vi "z_stack_waveform_Sunyee.vi"() -> ()   [LabVIEW 2018]
uses:
  <resource>/objmgr/daqmx.rc
  <vilib>/Utility/error.llb/DialogType.ctl
  <vilib>/DAQmx/create/channels.llb/DAQmx Create Channel (AO-Voltage-Basic).vi
  <vilib>/DAQmx/configure/timing.llb/DAQmx Timing (Sample Clock).vi
  <vilib>/Waveform/WDTOps.llb/WDT Append Waveforms DBL.vi
  <vilib>/DAQmx/write.llb/DAQmx Write (Analog 1D Wfm NChan NSamp).vi
  <vilib>/DAQmx/write.llb/DAQmx Write (Digital 1D Wfm NChan NSamp).vi
  <vilib>/DAQmx/configure/trigger.llb/DAQmx Start Trigger (Time).vi
  <vilib>/DAQmx/create/channels.llb/DAQmx Create Channel (DO-Digital Output).vi
  <vilib>/DAQmx/configure/trigger.llb/DAQmx Start Trigger (Digital Edge).vi
panel:
  in  "Line(s)":tag="Dev1/port0/line0:7"
  in  "Stop 2":bool
  in  "Trigger Type":T1(tab)
  in  "Edge":i32(ring)=10280 items=["Rising"=10280, "Falling"=10171]
  in  "Digital Trigger Source":tag="PFI1"
  in  "When":timestamp
  in  "Select Time\nManually":bool
  in  "Number of Samples":i32=1000
  in  "Sample Rate 2":dbl=1000.0
  in  "Sample Clock Source 2":tag="PFI0"
  out "Actual Sample Rate 2":dbl=1000.0 format="%0.2f"
  out "Waveform Graph 3":waveform(dbl)(graph)
  out "Waveform Graph 2":waveform(dbl)(graph)
  out "Waveform Graph":waveform(dbl)[](graph)
  in  "Stop":bool
  in  "Sample Rate":dbl=50000.0
  in  "Sample Clock Source":tag="OnboardClock"
  in  "Max Voltage":dbl=10.0
  in  "Min Voltage":dbl=-10.0
  in  "Physical Channel(s)":tag="PXI1Slot4_2/ao0:7"
  out "Actual Sample Rate":dbl=1000.0 format="%0.2f"
  # "To configure and use a start trigger you must have the necessary tab selected above.  Not all hardware supports triggering--refer to your device documentation for more info."
  # "If time is not manually set, task will begin after 10 seconds"
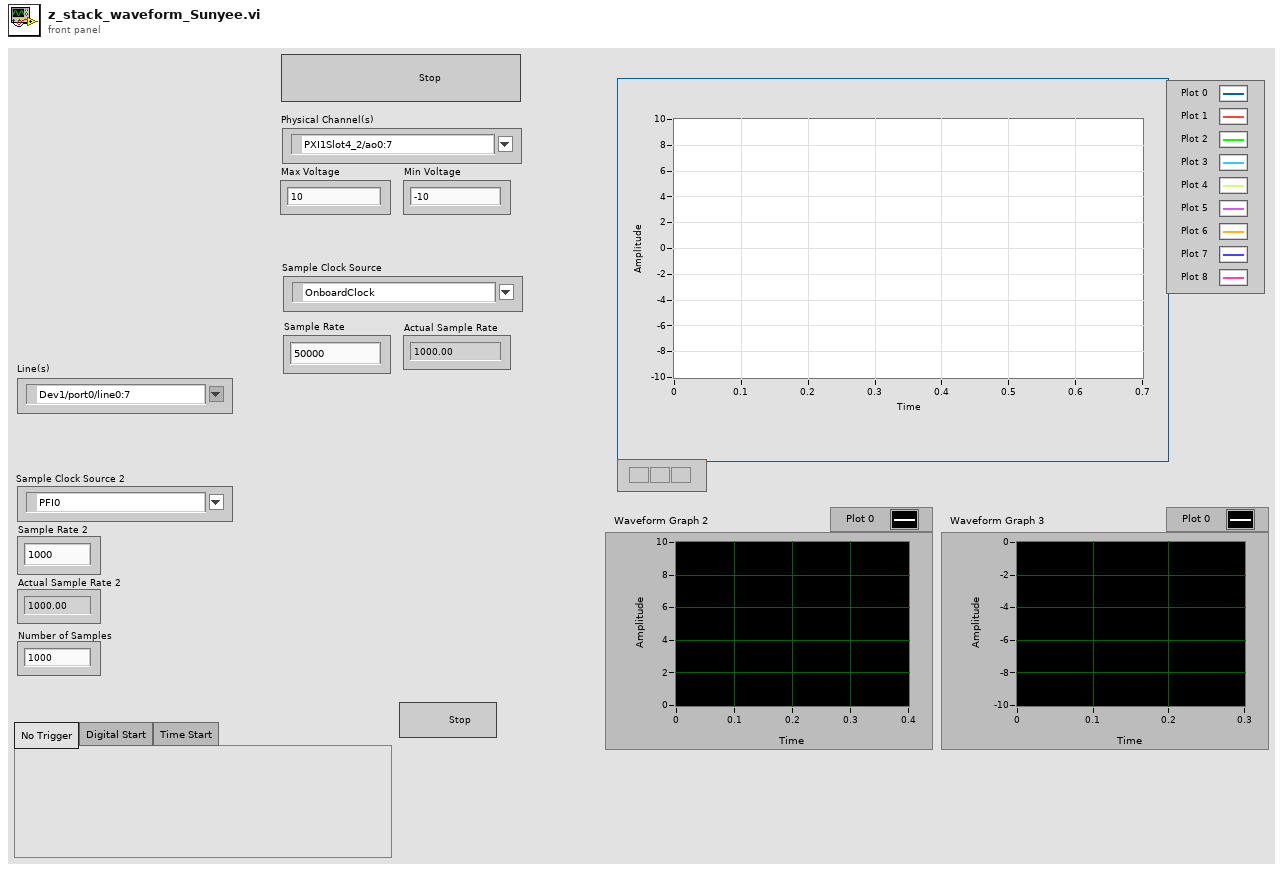
[diagram p1: front panel]
types:
  T1 = enum32{"No Trigger", "Digital Start", "Time Start"}
  T2 = typedef "DialogType.ctl" = u16
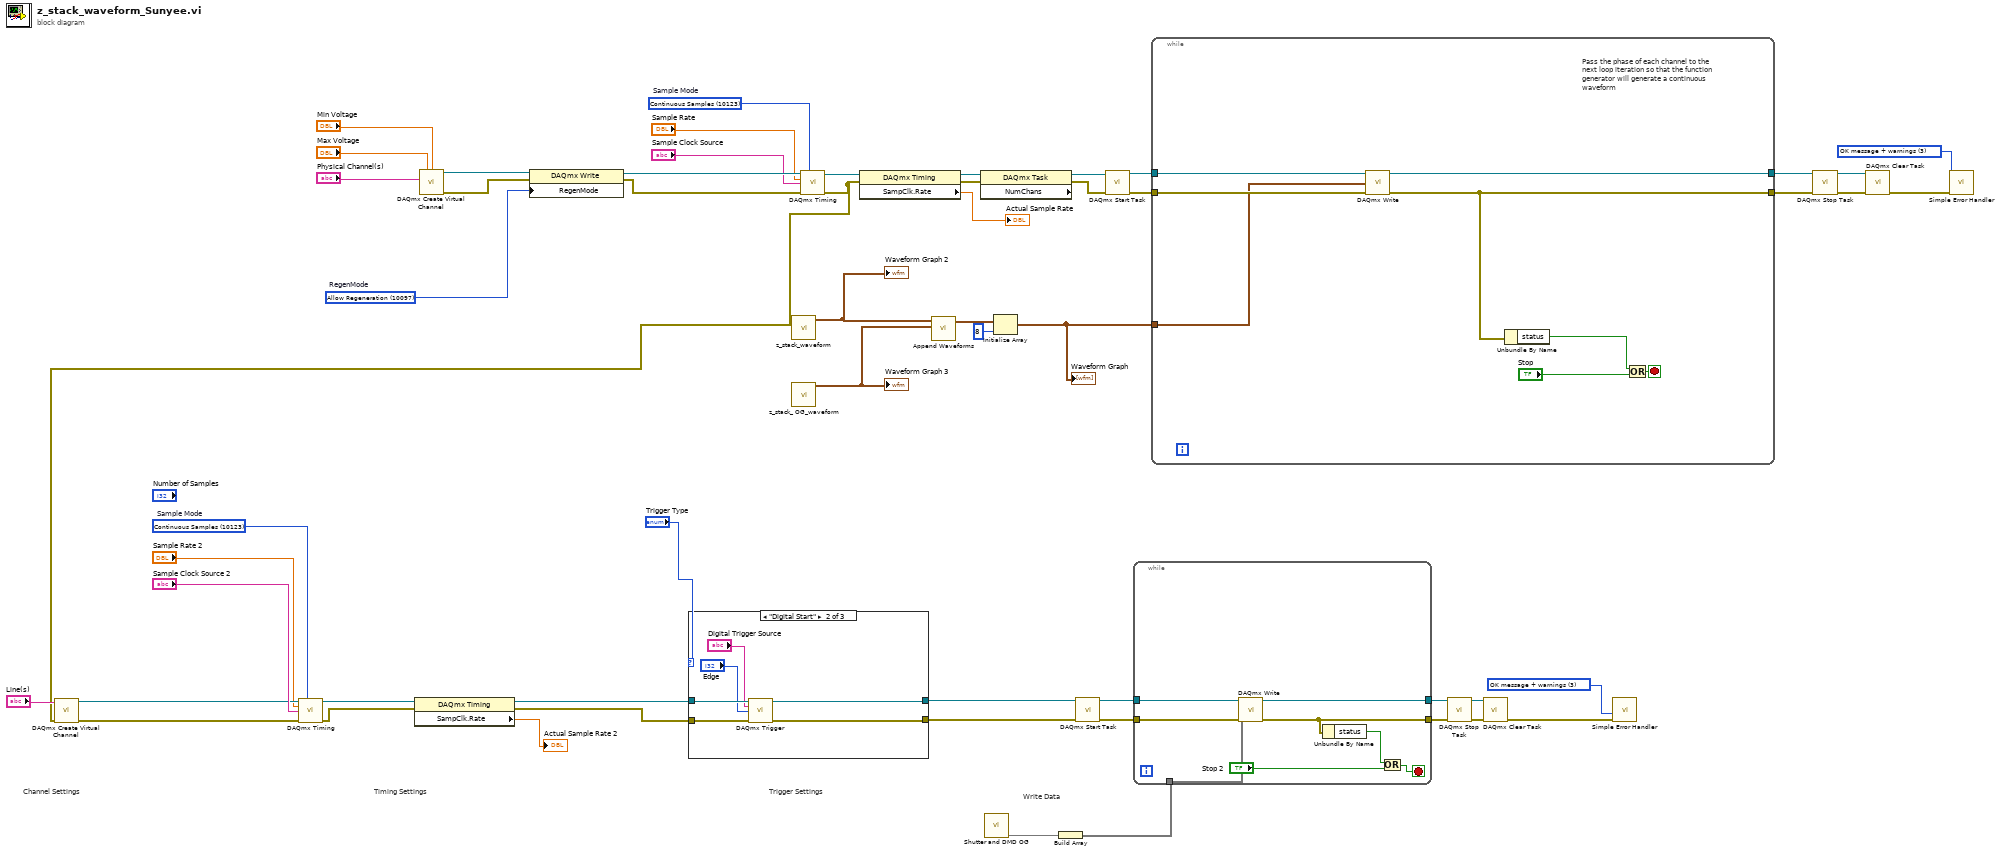
[diagram p0: block diagram]
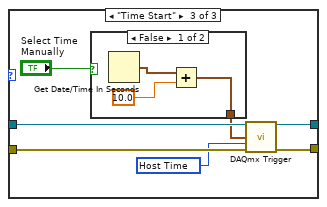
[diagram p3: hidden frame]
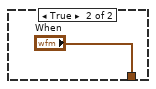
[diagram p4: hidden frame]
diagram:
  w6 = T2 3 items=["no dialog", "OK message", "continue or stop message", "OK message + warnings", "continue/stop + warnings"] ("type of dialog (OK msg:1)")
  w19 = 10123 items=["Finite Samples"=10178, "Continuous Samples"=10123, "Hardware Timed Single Point"=12522]  # Sample Mode
  w45 = T2 3 items=["no dialog", "OK message", "continue or stop message", "OK message + warnings", "continue/stop + warnings"] ("type of dialog (OK msg:1)")
  w51 = 10097 items=["Allow Regeneration"=10097, "Do Not Allow Regeneration"=10158]  # RegenMode
  w37 = 10123 items=["Finite Samples"=10178, "Continuous Samples"=10123, "Hardware Timed Single Point"=12522]  # Sample Mode
  # "Trigger Settings"
  # "Timing Settings"
  # "Write Data"
  # "Channel Settings"
  n1 = call-poly <vilib>:"DAQmx Create Virtual Channel.vi"("maximum value"="Max Voltage", "minimum value"="Min Voltage", "physical channels"="Physical Channel(s)") -> ("task out"=w53:refnum<k21>, "error out"=w52:errorcluster)  [unwired: 11 in]
  n2 = property class="DAQmx Write"(reference=w53, error in=w52, "RegenMode"=w51) -> (reference out=w50:refnum<k21>, error out=w34:errorcluster)
  n3 = call "z_stack_waveform.vi"() -> ("WaveformOut"=w31:waveform(dbl))  [unwired: 11 in]
  "Waveform Graph 2" <- w31
  n4 = call "z_stack_ OG_waveform.vi"() -> ("waveform out"=w30:waveform(dbl))  [unwired: 15 in, 4 out]
  "Waveform Graph 3" <- w30
  n5 = call-poly <vilib>:"DAQmx Timing.vi"("task/channels in"=w50, "sample mode"=w37, "rate"="Sample Rate", "source"="Sample Clock Source", "error in"=w34) -> ("task out"=w40:refnum<k21>, "error out"=w1:errorcluster)  [unwired: 9 in]
  n6 = call-poly <vilib>:"DAQmx Create Virtual Channel.vi"("lines"="Line(s)", "error in"=w1) -> ("task out"=w22:refnum<k21>, "error out"=w21:errorcluster)  [unwired: 12 in]
  n7 = call-poly <vilib>:"DAQmx Timing.vi"("task/channels in"=w22, "sample mode"=w19, "rate"="Sample Rate 2", "source"="Sample Clock Source 2", "error in"=w21) -> ("task out"=w18:refnum<k21>, "error out"=w17:errorcluster)  [unwired: 9 in]
  n8 = property class="DAQmx Timing"(reference=w18, error in=w17) -> (reference out=w15:refnum<k21>, error out=w14:errorcluster, "SampClk.Rate"=→"Actual Sample Rate 2":dbl)
  n9 = case shown="\"Digital Start\"" "Trigger Type" {
    tunnel: w15 -> [w57 w63 w70]
    tunnel: w14 -> [w56 w62 w69]
    tunnel: [w57 w61 w68] -> w5
    tunnel: [w56 w60 w67] -> w4
    frame "No Trigger", Default {
    }
    frame "Digital Start" {
      n10 = call-poly <vilib>:"DAQmx Trigger.vi"("task/channels in"=w63, "source"="Digital Trigger Source", "edge"="Edge", "error in"=w62) -> ("task out"=w61:refnum<k21>, "error out"=w60:errorcluster)  [unwired: 10 in]
    }
    frame "Time Start" {
      w64 = 16126 items=["Host Time"=16126, "I/O Device Time"=16127] ("timescale")
      n11 = case shown="False" "Select Time\nManually" {
        tunnel: [w72 "When"] -> w65
        frame False {
          n12 = Get Date/Time In Seconds() -> (seconds since 1Jan1904=w73:timestamp)
          n13 = Add(x=w73, y=10.0) -> (x+y=w72:timestamp)
        }
        frame True {
        }
      }
      n14 = call-poly <vilib>:"DAQmx Trigger.vi"("task/channels in"=w70, "when"=w65, "timescale"=w64, "error in"=w69) -> ("task out"=w68:refnum<k21>, "error out"=w67:errorcluster)  [unwired: 10 in]
    }
  }
  n15 = property class="DAQmx Timing"(reference=w40, error in=w1) -> (reference out=w44:refnum<k21>, error out=w43:errorcluster, "SampClk.Rate"=→"Actual Sample Rate":dbl)
  n16 = call-poly <vilib>:"Append Waveforms.vi"("waveform B"=w30, "waveform A"=w31) -> ("waveform out"=w28:waveform(dbl))  [unwired: 8 in, 1 out]
  n17 = property class="DAQmx Task" props=["NumChans"](reference=w44, error in=w43) -> (reference out=w26:refnum<k21>, error out=w33:errorcluster)  [unwired: 1 out]
  n18 = call "Shutter and DMD OG.vi"() -> (0:w3)  [unwired: 8 in, 2 out]
  n19 = Initialize Array(w28, 8 ("dimension size")) -> (w27:waveform(dbl)[])
  "Waveform Graph" <- w27
  n20 = Build Array(w3) -> (w2:void[])
  n21 = call <vilib>:"DAQmx Start Task.vi"("task/channels in"=w5, "error in"=w4) -> ("task out"=w13:refnum<k21>, "error out"=w12:errorcluster)  [unwired: 12 in]
  n22 = call <vilib>:"DAQmx Start Task.vi"("task/channels in"=w26, "error in"=w33) -> ("task out"=w41:refnum<k21>, "error out"=w42:errorcluster)  [unwired: 12 in]
  n23 = while {
    tunnel: w13 -> [w79]
    tunnel: w12 -> [w78]
    tunnel: [w77] -> w7
    tunnel: [w76] -> w8
    tunnel: w2 -> [w75]
    stop <- w80 stop-if-true
    n24 = call-poly <vilib>:"DAQmx Write.vi"("task/channels in"=w79, "data"=w75, "error in"=w78) -> ("task out"=w76:refnum<k21>, "error out"=w77:errorcluster)  [unwired: 10 in, 1 out]
    n25 = Unbundle By Name(w77) -> ("status"=w82:bool)
    n26 = Or(x=w82, y="Stop 2") -> (x .or. y?=w80:bool)
  }
  n27 = while {
    tunnel: w42 -> [w86]
    tunnel: [w84] -> w47
    tunnel: [w85] -> w46
    tunnel: w41 -> [w87]
    tunnel: w27 -> [w83]
    stop <- w89 stop-if-true
    # "Pass the phase of each channel to the next loop iteration so that the function generator will generate a continuous waveform"
    n28 = call-poly <vilib>:"DAQmx Write.vi"("task/channels in"=w87, "data"=w83, "error in"=w86) -> ("task out"=w84:refnum<k21>, "error out"=w85:errorcluster)  [unwired: 10 in, 1 out]
    n29 = Unbundle By Name(w85) -> ("status"=w88:bool)
    n30 = Or(x=w88, y="Stop") -> (x .or. y?=w89:bool)
  }
  n31 = call <vilib>:"DAQmx Stop Task.vi"("task/channels in"=w8, "error in"=w7) -> ("task out"=w10:refnum<k21>, "error out"=w9:errorcluster)  [unwired: 12 in]
  n32 = call <vilib>:"DAQmx Clear Task.vi"("task in"=w10, "error in"=w9) -> ("error out"=w25:errorcluster)  [unwired: 13 in]
  n33 = call <vilib>:"Simple Error Handler.vi"("type of dialog (OK msg:1)"=w6, "error in (no error)"=w25) -> ()  [unwired: 3 in, 5 out]
  n34 = call <vilib>:"DAQmx Stop Task.vi"("task/channels in"=w47, "error in"=w46) -> ("task out"=w49:refnum<k21>, "error out"=w48:errorcluster)  [unwired: 12 in]
  n35 = call <vilib>:"DAQmx Clear Task.vi"("task in"=w49, "error in"=w48) -> ("error out"=w55:errorcluster)  [unwired: 13 in]
  n36 = call <vilib>:"Simple Error Handler.vi"("type of dialog (OK msg:1)"=w45, "error in (no error)"=w55) -> ()  [unwired: 3 in, 5 out]
